vi "Averaged_Rot_Measure_Main_v3_gradient_comp - Copy.vi"() -> ()   [LabVIEW 2021]
uses:
  Config_File_Paths.ctl
  ZI_Data.ctl
  <vilib>/Analysis/baseanly.llb/Mean (DBL).vi
  <vilib>/Utility/file.llb/Write Delimited Spreadsheet (DBL).vi
  <vilib>/measure/maspectr.llb/FFT Spectrum (Real-Im) for 1 Chan.vi
  <vilib>/Analysis/NI_AALPro.lvlib
  <vilib>/measure/NI_MAPro.lvlib
  <vilib>/Analysis/NI_AALBase.lvlib
panel:
  out "phi":dbl
  out "Array 2":dbl[](array[numeric])
  out "Waveform Graph 3":waveform(dbl)[](graph)
  out "single differ 3":cluster{"Time":dbl[], "X":dbl[]}[](graph)
  out "output array":dbl[][](array[numeric])
  out "Waveform Graph 2":waveform(dbl)(graph)
  out "Array":dbl[](array[numeric])
  out "Waveform Graph":waveform(dbl)[](graph)
  out "Possible Mismatch In Phase (?)":bool
  out "Enough Points (?)":bool
  out "Trig Out Found(?)":bool
  out "Meter":dbl(knob) scale=-15.0..15.0
  out "single abs\nspectrum":waveform(dbl)(graph)
  out "single rot \nspectrum":waveform(dbl)[](graph)
  out "single differ":cluster{"Time":dbl[], "X":dbl[]}[](graph)
  out "single abs":cluster{"Time":dbl[], dbl[]}(graph)
  out "single rot":cluster{"Time":dbl[], "X":dbl[]}[](graph)
  in  "Resource Address":T1={"ZI Address"="DEV714", "VISA Keithley"="KEITHLEY", "VISA Arduino PG"="Arduino_PGen"}
  in  "error in":errorcluster
  in  "Config files paths":T2={"ZI config file (.ini)"="Config_Ver_1\\Zurich_params.ini", "Keithley config file (.ini)"="Config_Ver_1\\Keithley_params.ini", "Arduino config file (.ini)"="Config_Ver_1\\pulse_sequence.ini"}
  in  "Time unit":string(combo)="ms"
  out "loading":dbl(slide) scale=0.0..100.0
  in  "Number of averages":i32=1
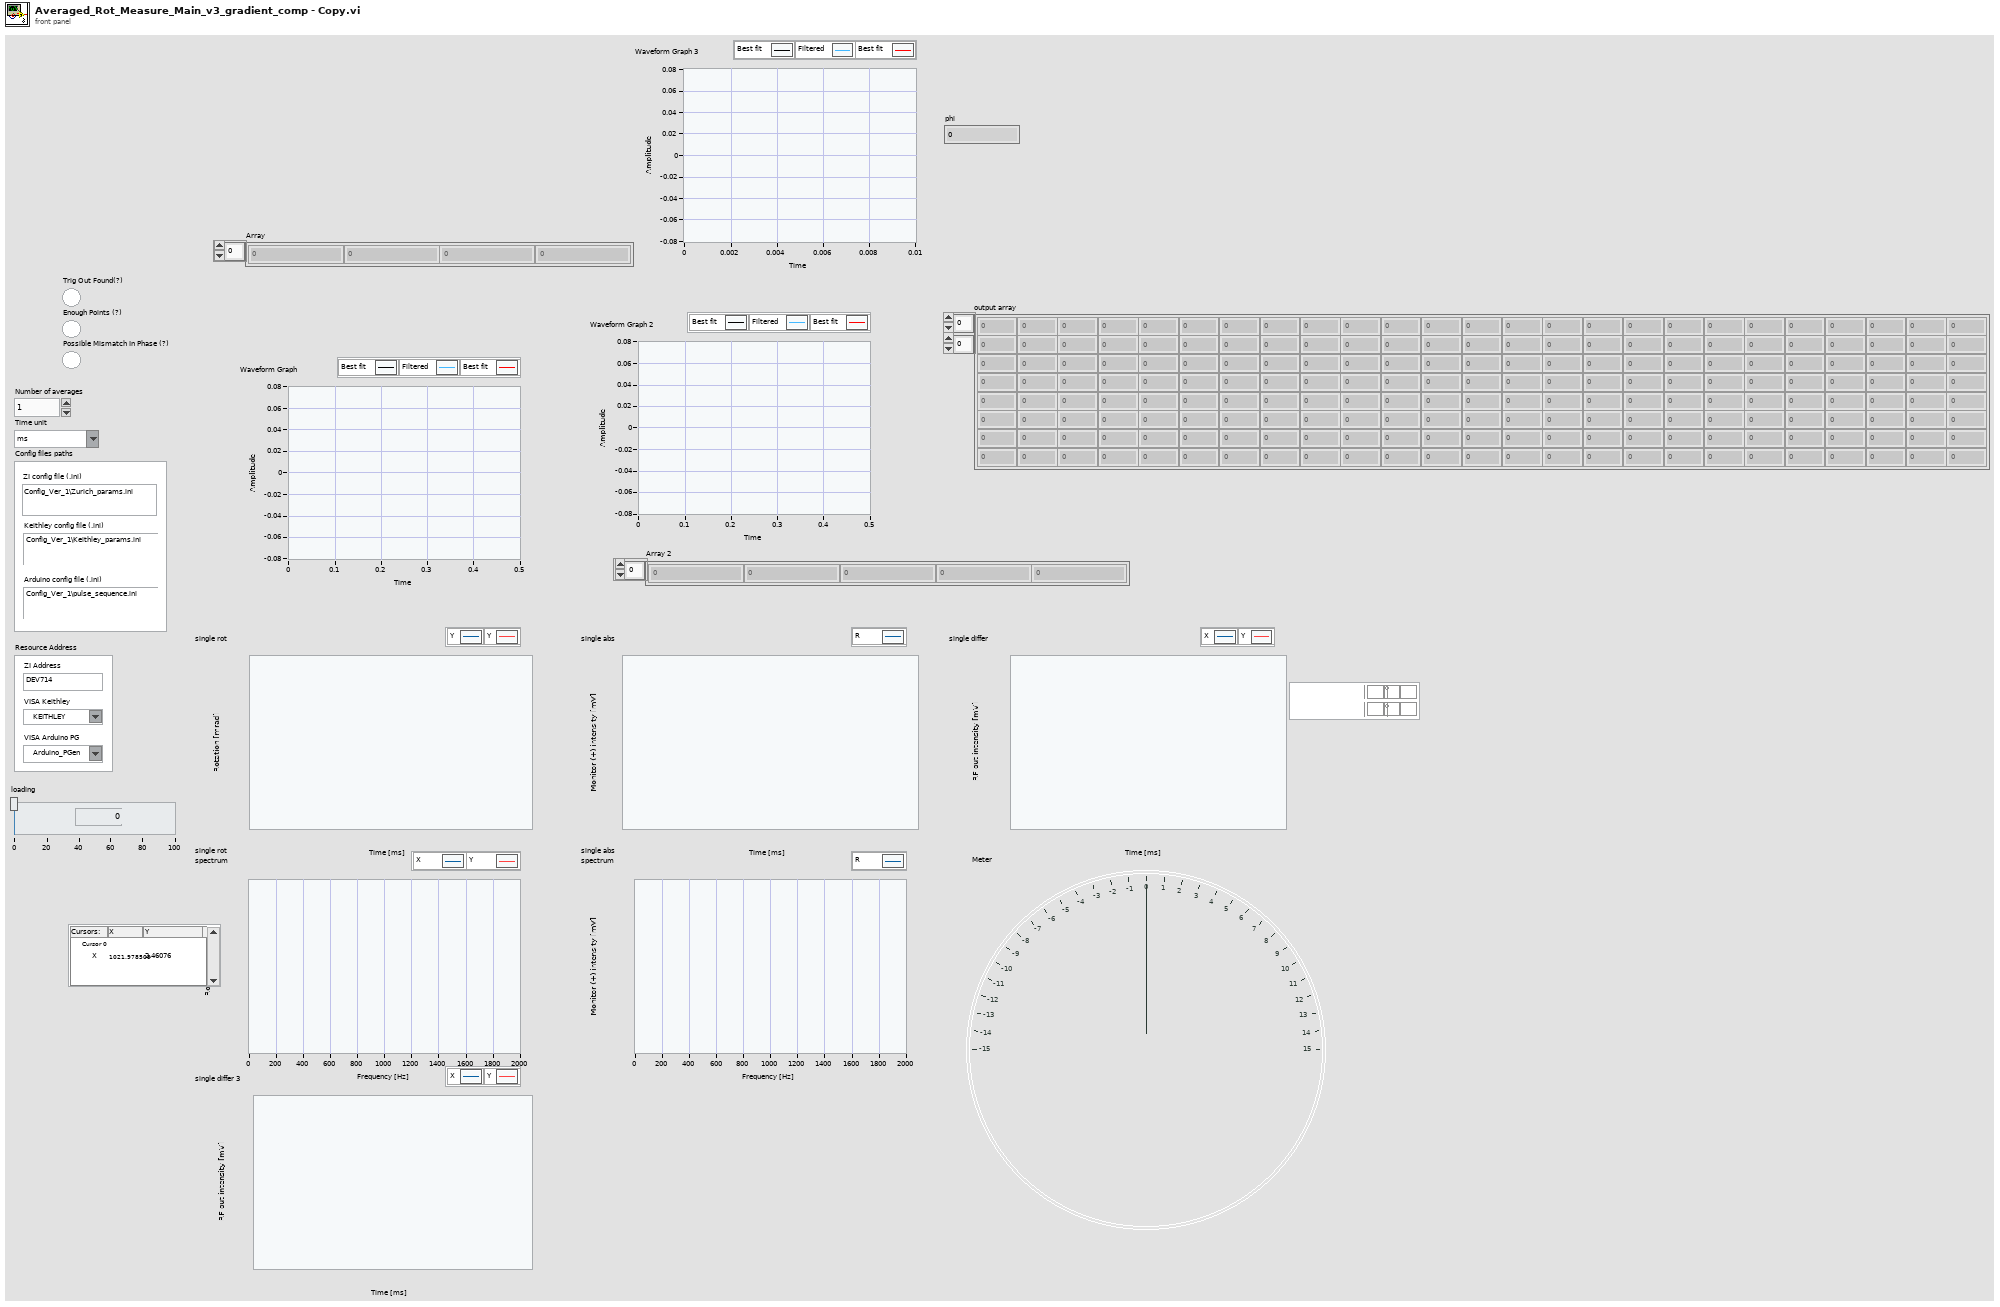
[diagram p1: front panel]
types:
  T1 = cluster{"ZI Address":string, "VISA Keithley":refnum<visa-resource-name>, "VISA Arduino PG":refnum<visa-resource-name>}
  T2 = typedef "Config_File_Paths.ctl" = cluster{"ZI config file (.ini)":string, "Keithley config file (.ini)":string, "Arduino config file (.ini)":string}
  T3 = typedef "ZI_Data.ctl" = cluster{"R":dbl[], "Theta":dbl[], "X":dbl[], "Y":dbl[], "AuxIn0":dbl[], "AuxIn1":dbl[], "Frequency":dbl[], "DIO":dbl[], "Time":dbl[]}
  T4 = typedef "Resources.ctl" = cluster{"ZI Handle":T5, "ZI ModHandle":T6, "VISA arduino":refnum<visa-resource-name>, "VISA Keithley":refnum<visa-resource-name>}
  T5 = typedef "Zurich Instruments LabOne.lvlib/ziTypeHandle.ctl" = cluster{"handleValid":bool, "Conn":u64, "Path Prefix":string, "Handle":u64, "Connected":bool, "Clockbase(s)":dbl}
  T6 = typedef "Zurich Instruments LabOne.lvlib/ziTypeModHandle.ctl" = cluster{"handleValid":bool, "Conn":u64, "ModHandle":u64, "moduleID":string, "Path Prefix":string}
  T7 = typedef "Cutted_Data.ctl" = cluster{"X":dbl[], "Y":dbl[], "Time":dbl[]}
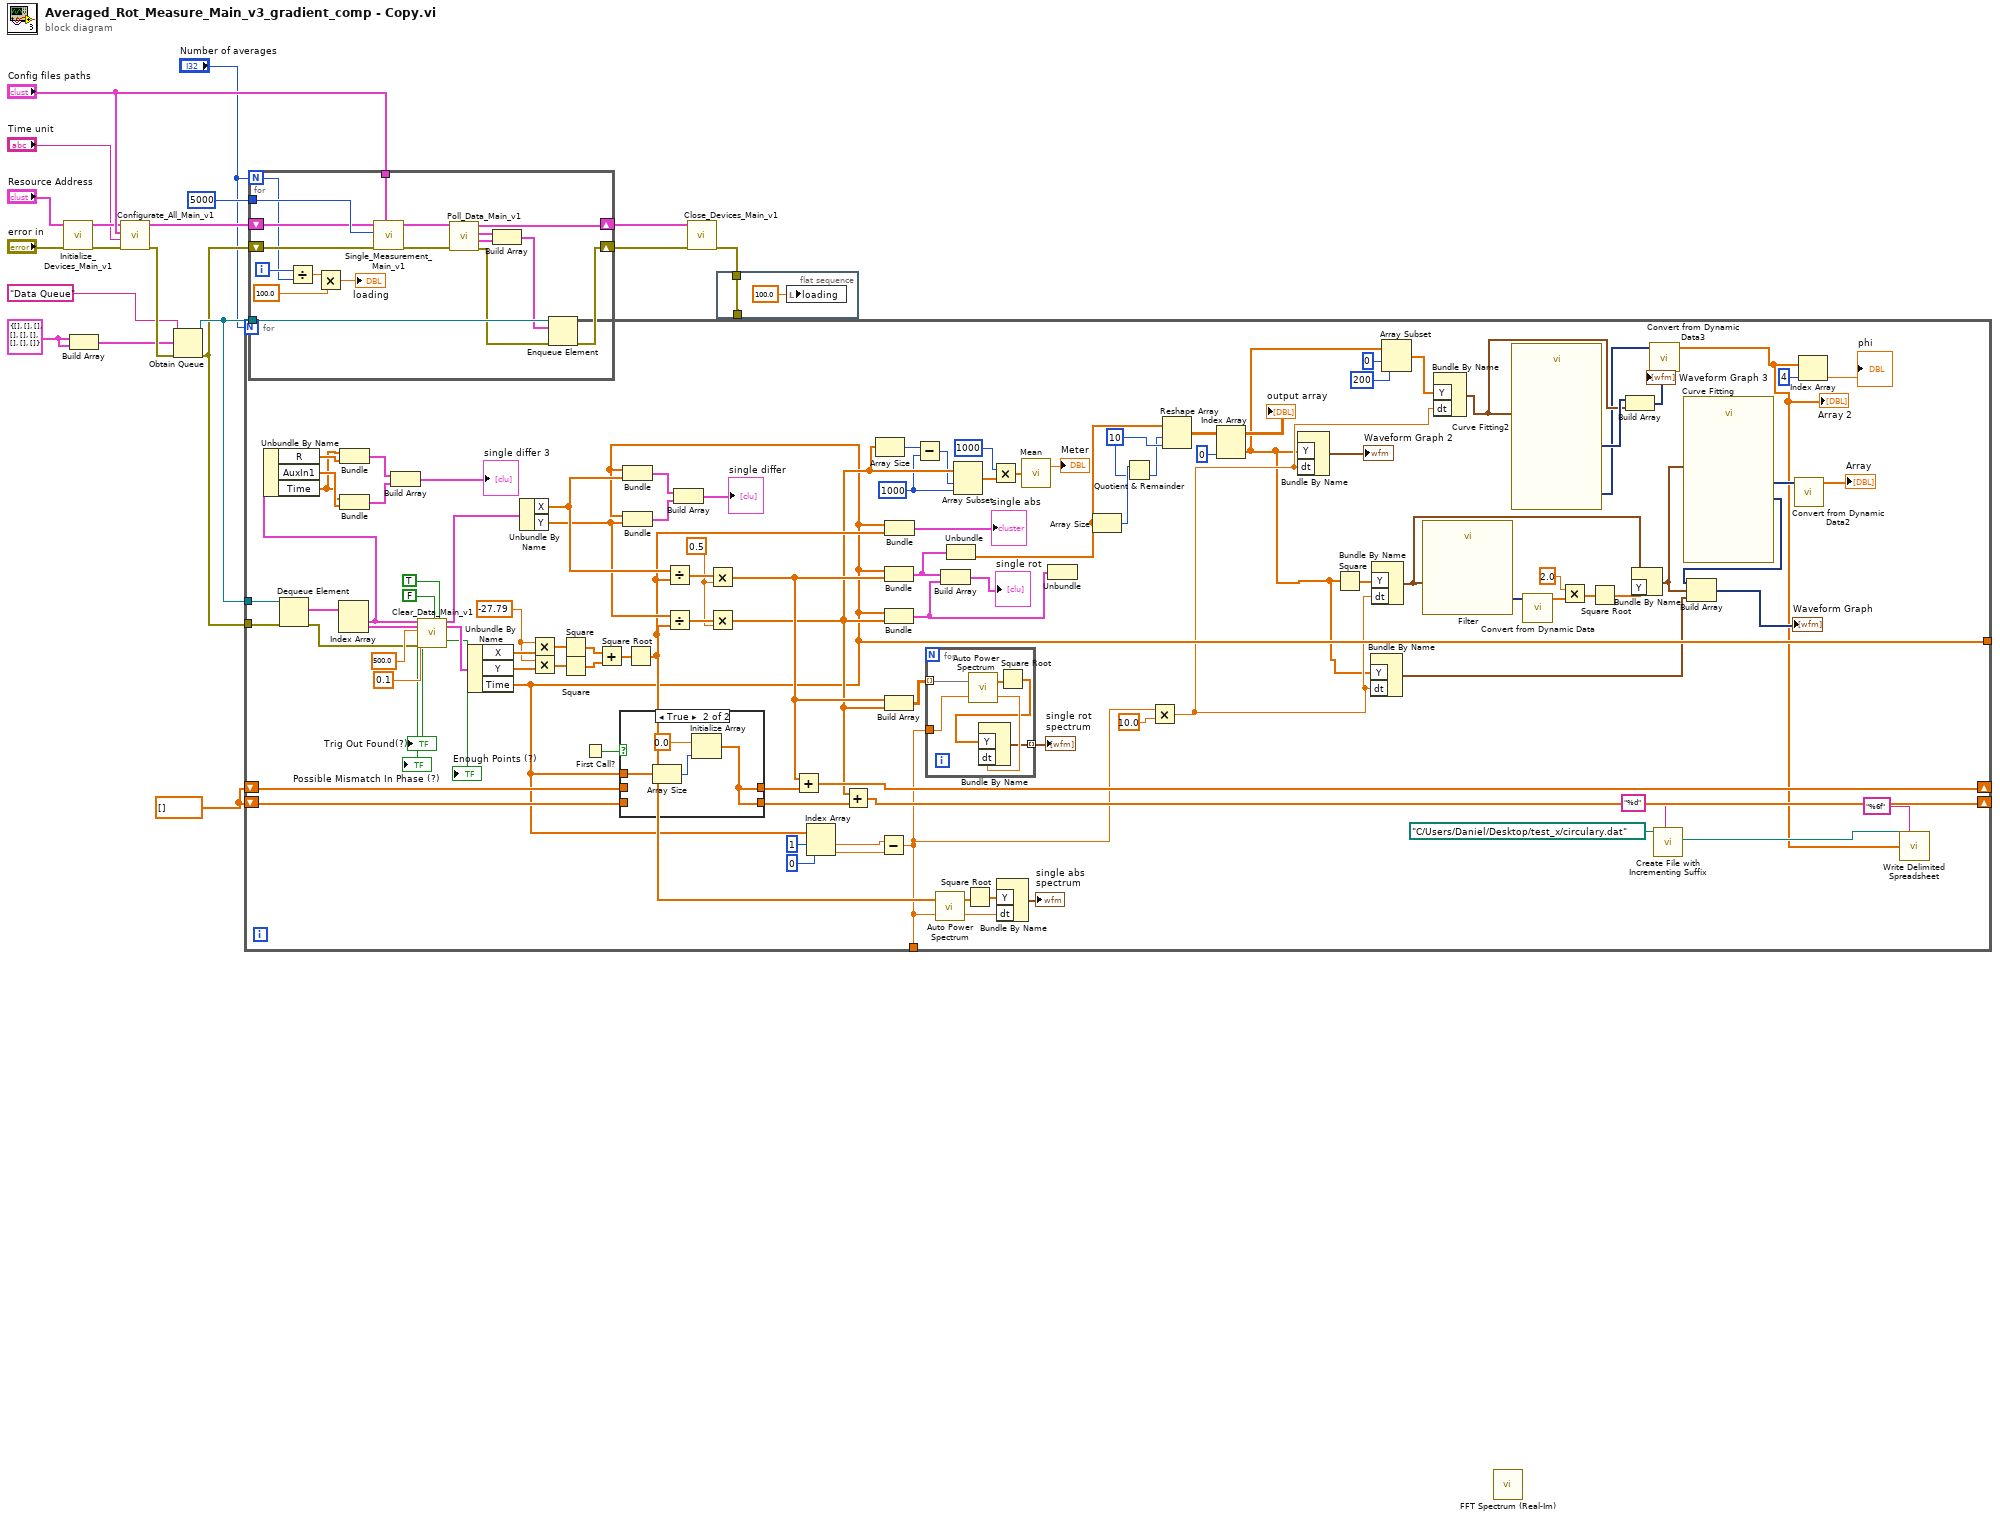
[diagram p0: block diagram]
diagram:
  w3 = dbl[] []
  w7 = T3 {"R"=[], "Theta"=[], "X"=[], "Y"=[], "AuxIn0"=[], "AuxIn1"=[], "Frequency"=[], "DIO"=[], "Time"=[]} ("ZI Data")
  n1 = call "Initialize_Devices_Main_v1.vi"("error in"="error in", "Resource Address"="Resource Address") -> ("error out"=w11:errorcluster, "Resources"=w12:T4)  [unwired: 8 in]
  n2 = Build Array(w7, w7) -> (w6:T3[])
  n3 = call "Configurate_All_Main_v1.vi"("error in"=w11, "Time unit"="Time unit", "Config files paths"="Config files paths", "Resources in"=w12) -> ("error out"=w9:errorcluster, "Resources out"=w17:T4)  [unwired: 4 in, 2 out]
  n4 = Obtain Queue(name (unnamed)="Data Queue", element data type=w6, error in (no error)=w9) -> (queue out=w5:refnum<queue>, error out=w4:errorcluster)  [unwired: 2 in, 1 out]
  n5 = for {
    N: "Number of averages" -> [_]
    tunnel: w5 -> [w126]
    tunnel: w4 -> [w125]
    shift-right: [w110] -> _
    shift-left: w3 -> [w114]
    shift-right: [w109] -> _
    shift-left: w3 -> [w113]
    tunnel: [w61] -> _
    tunnel: [w39] -> _
    w45 = 10 ("dimension size")
    w76 = 1000 ("length")
    w98 = 0.5
    w101 = -27.79
    n6 = Dequeue Element(queue=w126, error in (no error)=w125) -> (element=w124:T3[], error out=w120:errorcluster)  [unwired: 1 in, 2 out]
    n7 = Index Array(array=w124) -> (element #1=w67:T3, element #2=w123:T3)  [unwired: 2 in]
    n8 = Unbundle By Name(w67) -> ("R"=w64:dbl[], "AuxIn1"=w63:dbl[], "Time"=w62:dbl[])
    n9 = Bundle("Time"=w62, "R"=w64) -> (w66:cluster{"Time":dbl[], "R":dbl[]})  [unwired: 1 in]
    n10 = Bundle("Time"=w62, "AuxIn1"=w63) -> (w65:cluster{"Time":dbl[], "AuxIn1":dbl[]})  [unwired: 1 in]
    n11 = Build Array(w66, w65) -> (→"single differ 3":cluster{"Time":dbl[], "AuxIn1":dbl[]}[])
    n12 = call "Clear_Data_Main_v1.vi"("ZI Data 0"=w67, "ZI Data 3"=w123, "Time Of Collected Data (ms)"=500.0, "Crosstalk Tolerance"=0.1, "error in"=w120, "Fixed Number Of Points"=FALSE, "Check Phase Mismatch"=TRUE) -> ("Trig Out Found(?)"=→"Trig Out Found(?)":bool, "Enough Points (?)"=→"Enough Points (?)":bool, "Possible Mismatch In Phase (?)"=→"Possible Mismatch In Phase (?)":bool, "Cutted Data"=w117:T7, "Cutted Data 3"=w116:T7)  [unwired: 7 in, 1 out]
    n13 = Unbundle By Name(w116) -> ("X"=w102:dbl[], "Y"=w103:dbl[], "Time"=w61:dbl[])
    n14 = Unbundle By Name(w117) -> ("X"=w104:dbl[], "Y"=w91:dbl[])
    n15 = Multiply(x=w101, y=w102) -> (x*y=w87:dbl[])
    n16 = Multiply(x=w101, y=w103) -> (x*y=w86:dbl[])
    n17 = Square(x=w87) -> (x^2=w89:dbl[])
    n18 = Square(x=w86) -> (x^2=w88:dbl[])
    n19 = First Call?() -> (First Call?: T/F=w115:bool)
    n20 = Add(x=w89, y=w88) -> (x+y=w90:dbl[])
    n21 = case shown="True" w115 {
      tunnel: w61 -> [_ w138]
      tunnel: w114 -> [w134 _]
      tunnel: [w134 w135] -> w111
      tunnel: [w133 w135] -> w112
      tunnel: w113 -> [w133 _]
      frame False {
      }
      frame True {
        n22 = Array Size(array=w138) -> (size(s)=w136:i32)
        n23 = Initialize Array(0.0 ("element"), w136) -> (w135:dbl[])
      }
    }
    n24 = Bundle("Time"=w61, "X"=w104) -> (w107:cluster{"Time":dbl[], "X":dbl[]})  [unwired: 1 in]
    n25 = Bundle("Time"=w61, "Y"=w91) -> (w106:cluster{"Time":dbl[], "Y":dbl[]})  [unwired: 1 in]
    n26 = Square Root(x=w90) -> (sqrt(x)=w81:dbl[])
    n27 = Divide(x=w104, y=w81) -> (x/y=w100:dbl[])
    n28 = Divide(x=w91, y=w81) -> (x/y=w99:dbl[])
    n29 = Build Array(w107, w106) -> (→"single differ":cluster{"Time":dbl[], "Y":dbl[]}[])
    n30 = Multiply(x=w100, y=w98) -> (x*y=w84:dbl[])
    n31 = Multiply(x=w99, y=w98) -> (x*y=w77:dbl[])
    n32 = Add(x=w84, y=w111) -> (x+y=w110:dbl[])
    n33 = Index Array(array=w61, index #1=1 ("index"), index #2=0 ("index")) -> (element #1=w94:dbl, element #2=w93:dbl)
    n34 = Add(x=w77, y=w112) -> (x+y=w109:dbl[])
    n35 = Array Size(array=w77) -> (size(s)=w75:i32)
    n36 = Subtract(x=w94, y=w93) -> (x-y=w39:dbl)
    n37 = Bundle("Time"=w61, w84) -> (w21:cluster{"Time":dbl[], dbl[]})  [unwired: 1 in]
    n38 = Bundle("Time"=w61, w77) -> (w60:cluster{"Time":dbl[], dbl[]})  [unwired: 1 in]
    n39 = Build Array(w84, w77) -> (w97:dbl[][])
    n40 = Bundle("Time"=w61, w81) -> (→"single abs":cluster{"Time":dbl[], dbl[]})  [unwired: 1 in]
    n41 = Subtract(x=w75, y=w76) -> (x-y=w74:i32)
    n42 = for {
      tunnel: w97 -> [w132] mode=indexing
      tunnel: w39 -> [w131]
      tunnel: [w129] -> w92 mode=indexing
      n43 = call <vilib>:"Auto Power Spectrum.vi"("dt"=w131, "Signal (V)"=w132) -> ("df"=w130:dbl, "Power Spectrum (V^2 rms)"=w128:dbl[])
      n44 = Square Root(x=w128) -> (sqrt(x)=w127:dbl[])
      n45 = Bundle By Name("Y"=w127, "dt"=w130) -> (w129:waveform(dbl))  [unwired: 1 in]
    }
    "single rot \nspectrum" <- w92
    n46 = call <vilib>:"Auto Power Spectrum.vi"("dt"=w39, "Signal (V)"=w81) -> ("df"=w82:dbl, "Power Spectrum (V^2 rms)"=w83:dbl[])
    n47 = Build Array(w21, w60) -> (→"single rot":cluster{"Time":dbl[], dbl[]}[])
    n48 = Unbundle(w21) -> (w20:dbl[])  [unwired: 1 out]
    n49 = Array Subset(array=w77, index=w74, length=w76) -> (w73:dbl[])
    n50 = Square Root(x=w83) -> (sqrt(x)=w80:dbl[])
    n51 = Multiply(x=1000, y=w73) -> (x*y=w71:dbl[])
    n52 = Bundle By Name("Y"=w80, "dt"=w82) -> (→"single abs\nspectrum":waveform(dbl))  [unwired: 1 in]
    n53 = call-poly <vilib>:"Mean.vi"("X"=w71) -> ("mean"=→"Meter":dbl)  [unwired: 1 out]
    n54 = Unbundle(w60) -> ()  [unwired: 2 out]
    n55 = Array Size(array=w20) -> (size(s)=w47:i32)
    n56 = Quotient & Remainder(x=w47, y=w45) -> (floor(x/y)=w44:i32)  [unwired: 1 out]
    n57 = Multiply(x=w39, y=10.0) -> (x*y=w38:dbl)
    n58 = Reshape Array(w20, w44, w45) -> (w42:dbl[][])
    "output array" <- w42
    n59 = Index Array(array=w42, index (col)=0 ("disabled index (col)")) -> (element=w36:dbl[])  [unwired: 1 in]
    n60 = Bundle By Name("Y"=w36, "dt"=w38) -> (→"Waveform Graph 2":waveform(dbl))  [unwired: 1 in]
    n61 = Square(x=w36) -> (x^2=w48:dbl[])
    n62 = Bundle By Name("Y"=w36, "dt"=w38) -> (w40:waveform(dbl))  [unwired: 1 in]
    n63 = Bundle By Name("Y"=w48, "dt"=w38) -> (w55:waveform(dbl))  [unwired: 1 in]
    n64 = Array Subset(array=w36, index=0, length=200) -> (w33:dbl[])
    n65 = call "Filter"("Signal"=w55) -> ("Filtered Signal"=w58:dynamicdata)  [unwired: 9 in, 1 out]
    n66 = Bundle By Name("Y"=w33, "dt"=w38) -> (w31:waveform(dbl))  [unwired: 1 in]
    n67 = call "Curve Fitting2"("Signals"=w31) -> ("best fit"=w32:dynamicdata, "non-linear coefficients"=w29:dynamicdata)  [unwired: 6 in, 3 out]
    n68 = call "Convert from Dynamic Data"("Dynamic Data Type"=w58) -> ("Array"=w57:dbl[])  [unwired: 3 in]
    n69 = Multiply(x=2.0, y=w57) -> (x*y=w54:dbl[])
    n70 = Square Root(x=w54) -> (sqrt(x)=w53:dbl[])
    n71 = Build Array(w32, w31) -> (→"Waveform Graph 3":dynamicdata[])
    n72 = Bundle By Name(cluster=w55, "Y"=w53) -> (w41:waveform(dbl))
    n73 = call "Convert from Dynamic Data3"("Dynamic Data Type"=w29) -> ("Array"=w22:dbl[])  [unwired: 3 in]
    "Array 2" <- w22
    n74 = call <vilib>:"Create File with Incrementing Suffix.vi"("format string (\" (%d)\")"="%d" ("format string (\" (%d)\")"), "file path"=path "C:/Users/Daniel/Desktop/test_x/circulary.dat") -> ("actual path"=w24:path)  [unwired: 7 in, 2 out]
    n75 = call "Curve Fitting"("Signals"=w41) -> ("best fit"=w52:dynamicdata, "non-linear coefficients"=w51:dynamicdata)  [unwired: 6 in, 3 out]
    n76 = Build Array(w52, w41, w40) -> (→"Waveform Graph":dynamicdata[])
    n77 = call "Convert from Dynamic Data2"("Dynamic Data Type"=w51) -> ("Array"=→"Array":dbl[])  [unwired: 3 in]
    n78 = Index Array(array=w22, index=4) -> (element=→"phi":dbl)
    n79 = call-poly <vilib>:"Write Delimited Spreadsheet.vi"("file path (dialog if empty)"=w24, "format (%.3f)"="%6f", "1D data"=w22) -> ()  [unwired: 11 in, 2 out]
  }
  n80 = for {
    N: "Number of averages" -> [w148]
    shift-right: [w150] -> w18
    shift-left: w17 -> [w154]
    shift-right: [w139] -> w19
    shift-left: w4 -> [w153]
    tunnel: "Config files paths" -> [w156]
    tunnel: u64 5000 ("Timeout [ms]") -> [w155]
    tunnel: w5 -> [w144]
    i -> [w149]
    n81 = Divide(x=w149, y=w148) -> (x/y=w147:dbl)
    n82 = Multiply(x=w147, y=100.0) -> (x*y=→"loading":dbl)
    n83 = call "Single_Measurement_Main_v1.vi"("Config files paths"=w156, "error in"=w153, "Timeout [ms]"=w155, "Resources In"=w154) -> ("error out"=w151:errorcluster, "Resources Out"=w152:T4)  [unwired: 6 in]
    n84 = call "Poll_Data_Main_v1.vi"("error in"=w151, "Resources in"=w152) -> ("error out"=w140:errorcluster, "ZI Data 3"=w142:T3, "ZI Data 0"=w143:T3, "Resources out"=w150:T4)  [unwired: 6 in]
    n85 = Build Array(w143, w142) -> (w141:T3[])
    n86 = Enqueue Element(queue=w144, element=w141, error in (no error)=w140) -> (error out=w139:errorcluster)  [unwired: 1 in, 2 out]
  }
  n87 = call "Close_Devices_Main_v1.vi"("error in"=w19, "Resources in"=w18) -> ("error out"=w1:errorcluster)  [unwired: 9 in]
  n88 = flat-sequence {
    tunnel: [w157] -> _
    tunnel: w1 -> [w157]
    frame #0 {
      n89 = local write "loading"(100.0 ("loading")) -> ()
    }
  }
  n90 = call-poly <vilib>:"FFT Spectrum (Real-Im).vi"() -> ()  [unwired: 7 in, 5 out]
